vi "Untitled 1.vi"() -> ()   [LabVIEW 2017]
uses:
  System.Speech
panel:
  in  "Select Mode":bool
  in  "Delay Time (s)":dbl=1.0
  in  "Enter Your Text":string
  in  "Enter The File Path":path
  # "SPEECH TO TEXT CONVERTER"
  # "For Typing"
  # "To Read from file"
  # "Thank you.\nThis is a project by :\n-Prince Kumar Verma  - 190130103091\n-Mini Singh   - 190130103111\n-Mansi Singh - 190130103110"
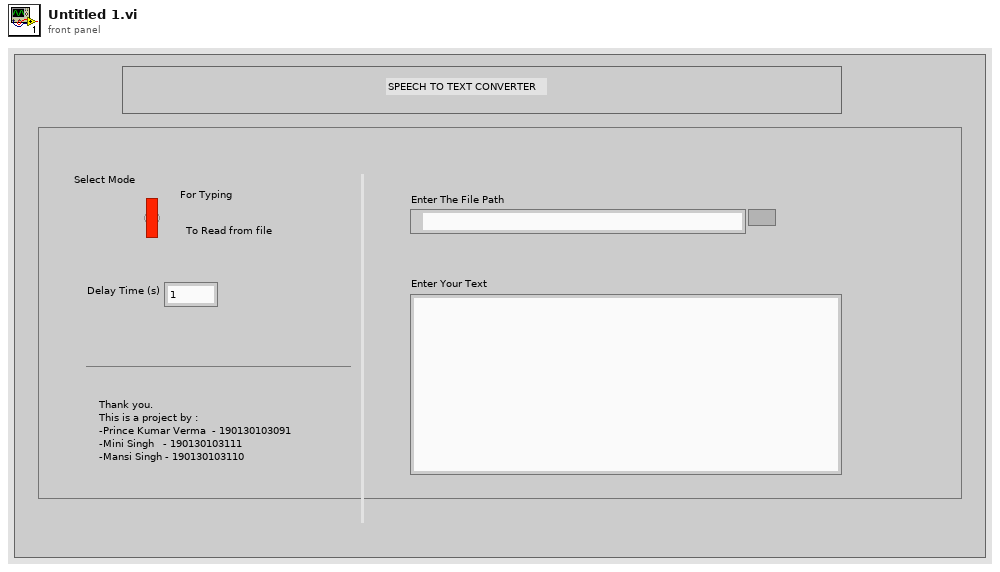
[diagram p1: front panel]
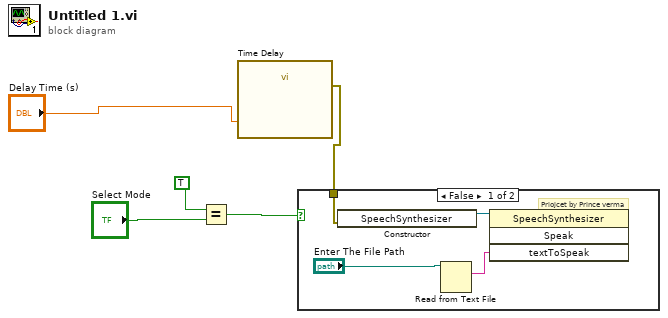
[diagram p0: block diagram]
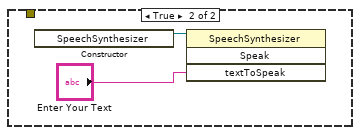
[diagram p2: hidden frame]
diagram:
  n1 = Equal?(x=TRUE, y="Select Mode") -> (x = y?=w4:bool)
  n2 = call "Time Delay"("Delay Time (s)"="Delay Time (s)") -> ("error out"=w3:errorcluster)  [unwired: 10 in]
  n3 = case shown="False" w4 {
    tunnel: w3 -> [w7 _]
    frame False {
      # "Priojcet by Prince verma"
      n4 = constructor class="SpeechSynthesizer"(error in=w7) -> (reference out=w8:refnum<k24>)  [unwired: 2 in, 2 out]
      n5 = Read from Text File(file (use dialog)="Enter The File Path") -> (text=w9:string)  [unwired: 3 in, 3 out]
      n6 = invoke class="SpeechSynthesizer" method="Speak"(reference=w8, "textToSpeak"=w9) -> ()  [unwired: 2 in, 4 out]
    }
    frame True {
      n7 = constructor class="SpeechSynthesizer"() -> (reference out=w11:refnum<k24>)  [unwired: 3 in, 2 out]
      n8 = invoke class="SpeechSynthesizer" method="Speak"(reference=w11, "textToSpeak"="Enter Your Text") -> ()  [unwired: 2 in, 4 out]
    }
  }
